vi "test joystick .vi"(11 "controller IN":T1) -> (3 "controller OUT":T1)   [LabVIEW 2016]
uses:
  Classes/Controller/Motion/A3200 Folder/A3200.lvclass
  Classes/Controller/Dispenser/Ultimus V2 Folder/Ultimus V2.lvclass
  Classes/Controller/I-O/NI-DAQ Folder/NI-DAQ.lvclass
  Classes/Controller/Motion/Motion Folder/Motion.lvclass
  Classes/Controller/I-O/I-O Folder/I-O.lvclass
  Classes/Controller/Dispenser/Dispenser Folder/Dispenser.lvclass
panel:
  out "XYZTheta Out":dbl[](array[numeric]) format="%#_8g"
  in  "Numeric":i32=1 min=1 max=500
  in  "stop":bool
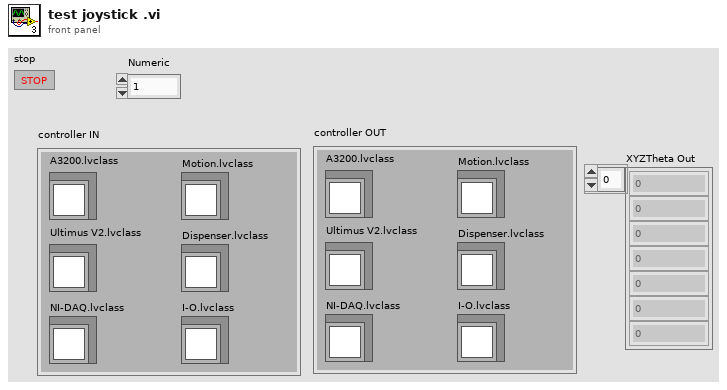
[diagram p1: front panel]
types:
  T1 = cluster{"A3200.lvclass":refnum<class "A3200.lvclass">, "Ultimus V2.lvclass":refnum<class "Ultimus V2.lvclass">, "NI-DAQ.lvclass":refnum<class "NI-DAQ.lvclass">, "Motion.lvclass":refnum<class "Motion.lvclass">, "I-O.lvclass":refnum<class "I-O.lvclass">, "Dispenser.lvclass":refnum<class "Dispenser.lvclass">}
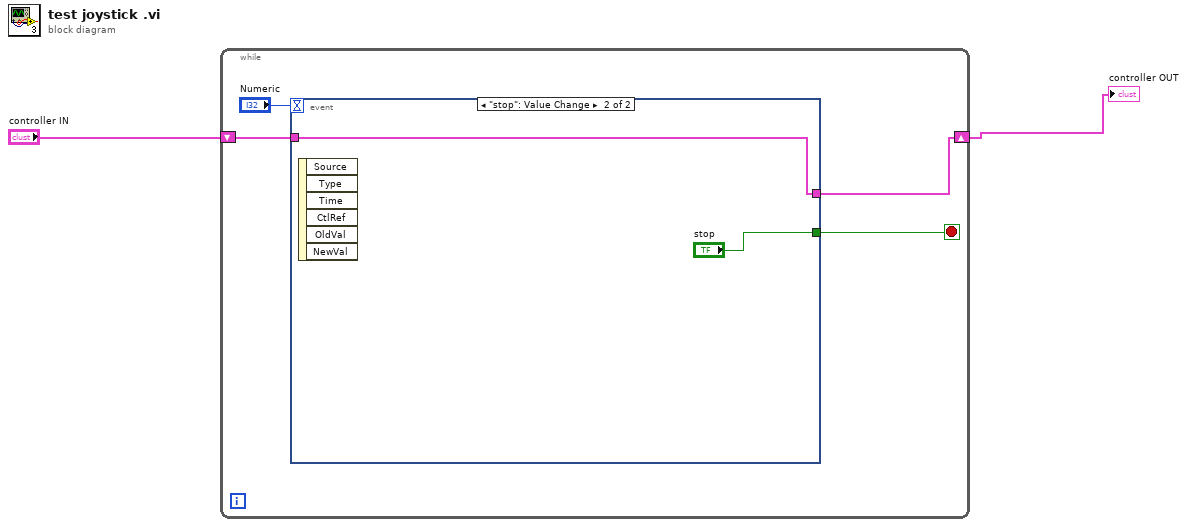
[diagram p0: block diagram]
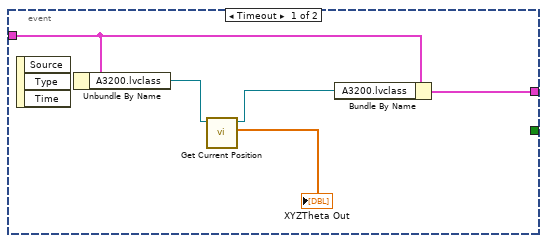
[diagram p2: hidden frame]
diagram:
  n1 = while {
    shift-right: [w3] -> w1
    shift-left: "controller IN" -> [w4]
    stop <- w6 stop-if-true
    n2 = event shown="[1] \"stop\": Value Change" {
      selector: _ -> [_ _]
      dyn-events: _ -> [_ _]
      timeout: "Numeric" -> [_ _]
      tunnel: [_ "stop"] -> w6
      tunnel: w4 -> [w11 w12]
      tunnel: [w10 w12] -> w3
      event Timeout {
        n3 = event-data() -> ()  [unwired: 1 in, 3 out]
        n4 = Unbundle By Name(w11) -> ("A3200.lvclass"=w9:refnum<class "A3200.lvclass">)
        n5 = call-dynamic "Get Current Position.vi"("Gantry in"=w9) -> ("XYZTheta Out"=→"XYZTheta Out":dbl[], "Gantry out"=w8:refnum<class "A3200.lvclass">)  [unwired: 8 in, 1 out]
        n6 = Bundle By Name(cluster=w11, "A3200.lvclass"=w8) -> (w10:T1)
      }
      event "stop": Value Change {
        n7 = event-data() -> ()  [unwired: 1 in, 6 out]
      }
    }
  }
  "controller OUT" <- w1
